vi "RateofChangeThermistor.vi"(10 "Last Reading":dbl[](array[numeric]), 11 "Current Reading":dbl[](array[numeric])) -> (3 "Rate of Change Output":dynamicdata(waveform))   [LabVIEW 2020]
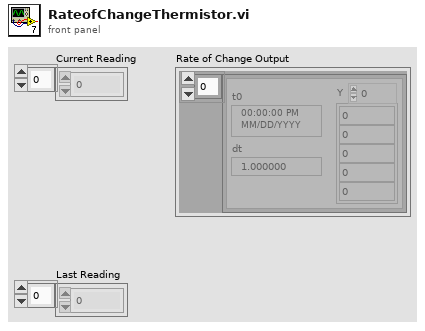
[diagram p1: front panel]
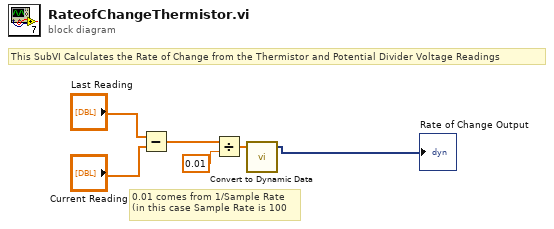
[diagram p0: block diagram]
diagram:
  # "0.01 comes from 1/Sample Rate\n(in this case Sample Rate is 100"
  # "This SubVI Calculates the Rate of Change from the Thermistor and Potential Divider Voltage Readings"
  n1 = Subtract(x="Last Reading", y="Current Reading") -> (x-y=w1:dbl[])
  n2 = Divide(x=w1, y=0.01) -> (x/y=w3:dbl[])
  n3 = call "Convert to Dynamic Data"("Array"=w3) -> ("Dynamic Data Type"=→"Rate of Change Output":dynamicdata)  [unwired: 3 in]
